vi "判别式.vi"(7 "A":dbl, 10 "C":dbl, 11 "B":dbl) -> (3 "判别式":dbl)   [LabVIEW 2018]
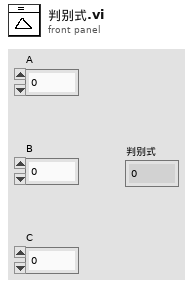
[diagram p1: front panel]
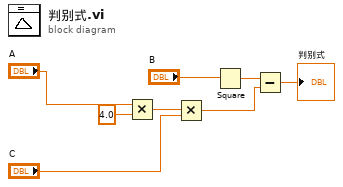
[diagram p0: block diagram]
diagram:
  n1 = Multiply(x="A", y=4.0) -> (x*y=w5:dbl)
  n2 = Multiply(x=w5, y="C") -> (x*y=w2:dbl)
  n3 = Square(x="B") -> (x^2=w3:dbl)
  n4 = Subtract(x=w3, y=w2) -> (x-y=→"判别式":dbl)
